vi "receive_photon_buffer.vi"(8 "error in (no error)":errorcluster, 11 "hydraharp in":refnum<class "hydraharp.lvclass">) -> (0 "error out":errorcluster, 2 "done?":bool, 3 "hydraharp out":refnum<class "hydraharp.lvclass">)   [LabVIEW 2015, in "hydraharp.lvclass"]
uses:
  hydraharp.lvclass
  hydraharp.lvclass/hydraharp.ctl
  hydraharp_fifo_queue_data.ctl
  hydraharp_fifo_actions.ctl
  hhlib.dll
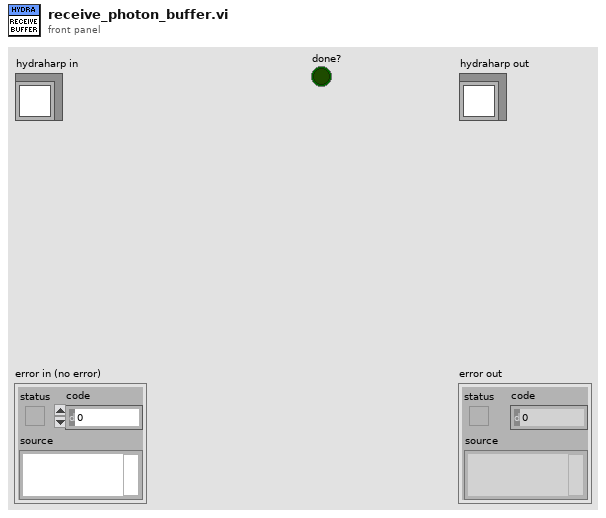
[diagram p1: front panel]
types:
  T1 = typedef "hydraharp_fifo_queue_data.ctl" = cluster{"fifo_buffer":u32[], "fifo_action":T2}
  T2 = typedef "hydraharp_fifo_actions.ctl" = enum16{"stop", "new_data"}
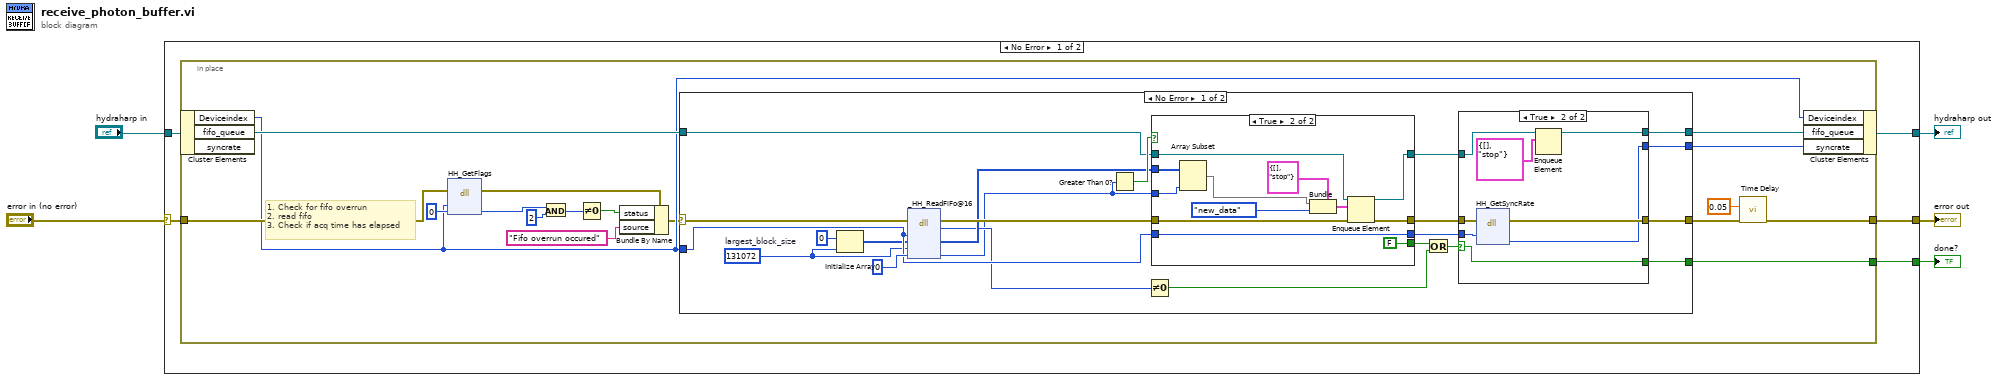
[diagram p0: block diagram]
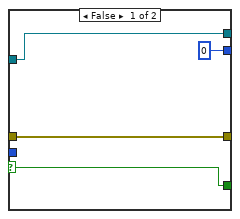
[diagram p2: hidden frame]
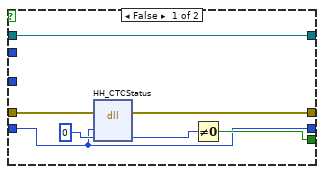
[diagram p3: hidden frame]
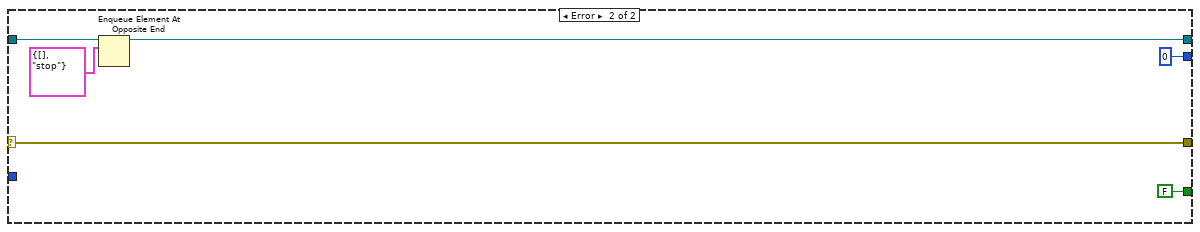
[diagram p4: hidden frame]
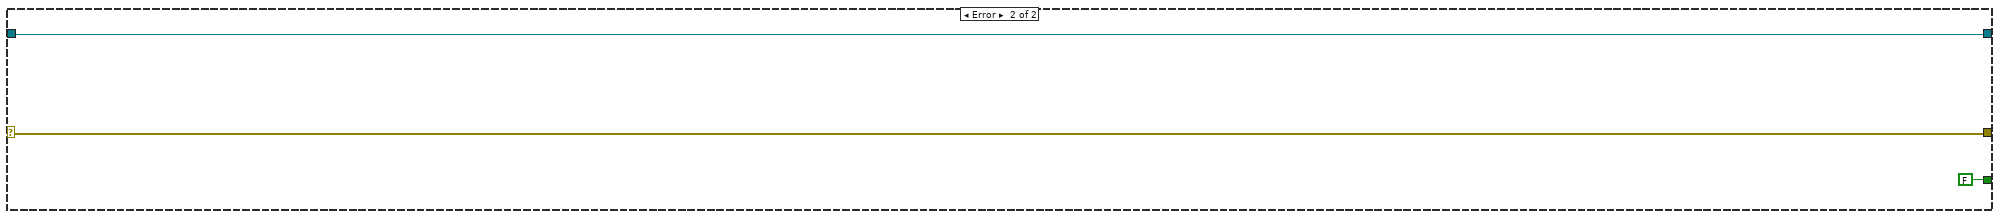
[diagram p5: hidden frame]
diagram:
  n1 = case shown="No Error" "error in (no error)" {
    selector: "error in (no error)" -> [w9 w89]
    tunnel: [w8 w89] -> w3
    tunnel: [w7 w88] -> w2
    tunnel: "hydraharp in" -> [w10 w88]
    tunnel: [w6 FALSE] -> w1
    frame No Error {
      n2 = in-place {
        in-place-border: w9 -> [w27]
        in-place-border: [w12] -> w8
        in-place-border: [w20] -> w6
        # "1. Check for fifo overrun\n2. read fifo\n3. Check if acq time has elapsed"
        n3 = in-place-cluster #1(w10) -> ("Deviceindex"=w21:i32, "fifo_queue"=w23:refnum<queue>)  [unwired: 1 out]
        n4 = dll-call lib="hhlib.dll" fn="HH_GetFlags"(error in=w27, "devidx"=w21, "flags"=0) -> (error out=w19:errorcluster, "flags"=w25:i32)  [unwired: 4 in, 1 out]
        n5 = And(x=w25, y=2) -> (x .and. y?=w16:i32)
        n6 = Not Equal To 0?(x=w16) -> (x != 0?=w15:bool)
        n7 = Bundle By Name(cluster=w19, "status"=w15, "source"="Fifo overrun occured") -> (w17:errorcluster)
        n8 = case shown="No Error" w17 {
          selector: w17 -> [w37 w82]
          tunnel: w21 -> [w46 _]
          tunnel: w23 -> [w44 w86]
          tunnel: [w40 w85] -> w22
          tunnel: [w39 w82] -> w13
          tunnel: [w38 FALSE] -> w20
          tunnel: [w28 0 ("syncrate")] -> w11
          frame No Error {
            w31 = 131072  # largest_block_size
            n9 = Initialize Array(u32 0 ("element"), w31) -> (w30:u32[])
            n10 = dll-call lib="hhlib.dll" fn="_HH_ReadFiFo@16" label="HH_ReadFiFo"(error in=w37, "devidx"=w46, "buffer"=w30, "blocksize"=w31, "nactual"=0) -> (error out=w47:errorcluster, "return type"=w36:i32, "buffer"=w43:u32[], "nactual"=w33:i32)  [unwired: 4 in, 1 out]
            n11 = Greater Than 0?(x=w33) -> (x > 0?=w48:bool)
            n12 = Not Equal To 0?(x=w36) -> (x != 0?=w35:bool)
            n13 = case shown="True" w48 {
              tunnel: w47 -> [w68 w78]
              tunnel: [w67 w73] -> w34
              tunnel: w46 -> [w62 w69]
              tunnel: [w64 FALSE] -> w45
              tunnel: w44 -> [w65 w79]
              tunnel: w43 -> [_ w72]
              tunnel: [w65 w74] -> w41
              tunnel: w33 -> [_ w70]
              tunnel: [w62 w69] -> w29
              frame False {
                n14 = dll-call lib="hhlib.dll" fn="HH_CTCStatus"(error in=w68, "devidx"=w62, "status"=0) -> (error out=w67:errorcluster, "status"=w63:i32)  [unwired: 4 in, 1 out]
                n15 = Not Equal To 0?(x=w63) -> (x != 0?=w64:bool)
              }
              frame True {
                n16 = Array Subset(array=w72, length=w70) -> (w71:u32[])  [unwired: 1 in]
                n17 = Bundle(cluster=T1 {"fifo_buffer"=[], "fifo_action"=enum."stop"} ("output cluster"), "fifo_buffer"=w71, "fifo_action"=hydraharp_fifo_actions."new_data") -> (w75:T1)
                n18 = Enqueue Element(queue=w79, element=w75, error in (no error)=w78) -> (queue out=w74:refnum<queue>, error out=w73:errorcluster)  [unwired: 1 in, 1 out]
              }
            }
            n19 = Or(x=w45, y=w35) -> (x .or. y?=w42:bool)
            n20 = case shown="True" w42 {
              selector: w42 -> [w51 w58]
              tunnel: w41 -> [w53 w61]
              tunnel: [w53 w59] -> w40
              tunnel: w34 -> [w52 w57]
              tunnel: [w52 w56] -> w39
              tunnel: [w51 w58] -> w38
              tunnel: w29 -> [_ w55]
              tunnel: [0 ("syncrate") w54] -> w28
              frame False {
              }
              frame True {
                n21 = dll-call lib="hhlib.dll" fn="HH_GetSyncRate"(error in=w57, "devidx"=w55) -> (error out=w56:errorcluster, "syncrate"=w54:i32)  [unwired: 5 in, 1 out]
                n22 = Enqueue Element(queue=w61, element=T1 {"fifo_buffer"=[], "fifo_action"=enum."stop"}) -> (queue out=w59:refnum<queue>)  [unwired: 2 in, 2 out]
              }
            }
          }
          frame Error {
            n23 = Enqueue Element At Opposite End(queue=w86, element=T1 {"fifo_buffer"=[], "fifo_action"=enum."stop"}) -> (queue out=w85:refnum<queue>)  [unwired: 2 in, 2 out]
          }
        }
        n24 = call "Time Delay"("error in (no error)"=w13, "Delay Time (s)"=0.05) -> ("error out"=w12:errorcluster)  [unwired: 9 in]
        n25 = in-place-cluster #1("Deviceindex"=w21, "fifo_queue"=w22, "syncrate"=w11) -> (w7:refnum<class "hydraharp.lvclass">)
      }
    }
    frame Error {
    }
  }
  "error out" <- w3
  "hydraharp out" <- w2
  "done?" <- w1
